vi "HandlesNullsInDB.vi"() -> ()   [LabVIEW 2019]
uses:
  <vilib>/Utility/error.llb/DialogType.ctl
  <vilib>/addons/database/Connection.llb/DB Tools Open Connec (String).vi
  <vilib>/addons/database/_DB Variant To Data/Database Variant To Data.xnode
  <vilib>/addons/database/NI_Database_API.lvlib
panel:
  out "Null Value Handled For  String":string[][](array[string])
  out "Original Data":string[][](array[string])
  out "With   Null Handled  for  Numeric":variant[][](array[variant])
  out "data":variant[][](array[variant])
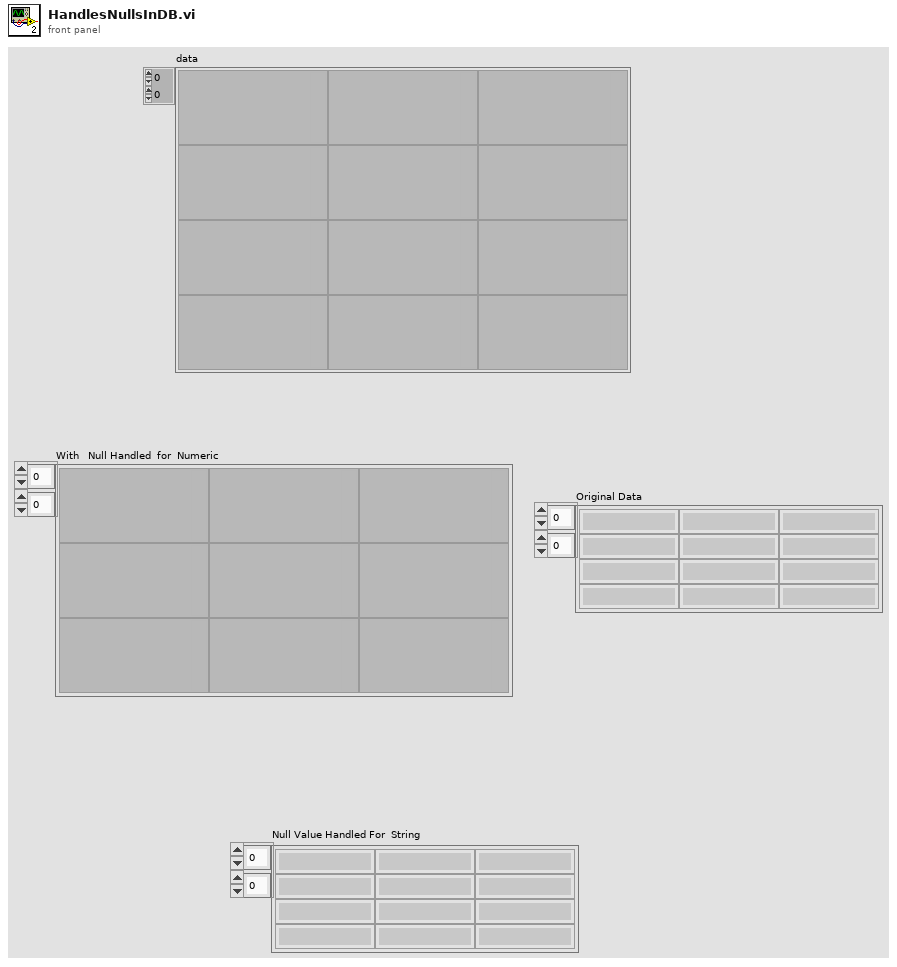
[diagram p1: front panel]
types:
  T1 = typedef "DialogType.ctl" = u16
  T2 = typedef "NI_Database_API.lvlib/Conn ObjectReference.ctl" = refnum<k1>
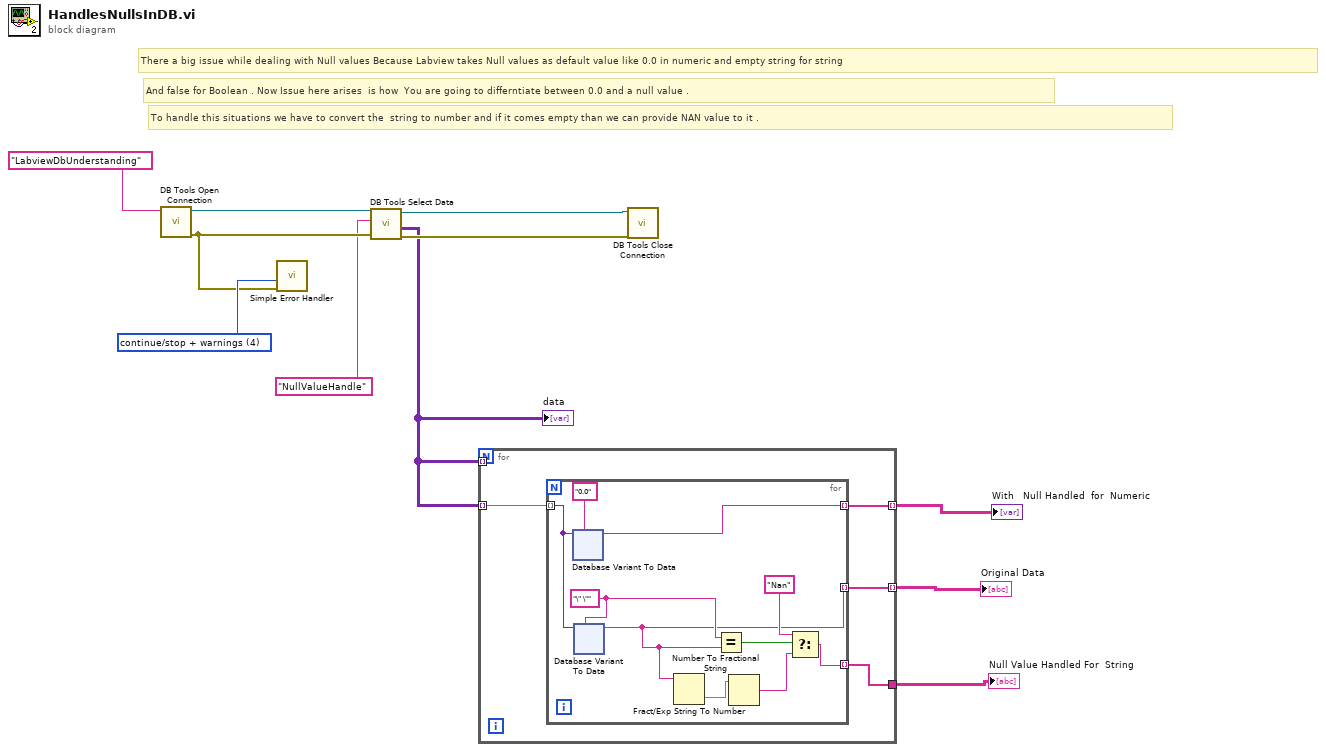
[diagram p0: block diagram]
diagram:
  w10 = T1 4 items=["no dialog", "OK message", "continue or stop message", "OK message + warnings", "continue/stop + warnings"] ("type of dialog (OK msg:1)")
  # "To handle this situations we have to convert the  string to number and if it comes empty than we can provide NAN value to it ."
  # "And false for Boolean . Now Issue here arises  is how  You are going to differntiate between 0.0 and a null value ."
  # "There a big issue while dealing with Null values Because Labview takes Null values as default value like 0.0 in numeric and empty string for string"
  n1 = call-poly <vilib>:"DB Tools Open Connection.vi"("connection information"="LabviewDbUnderstanding") -> ("error out"=w8:errorcluster, "connection reference"=w9:T2)  [unwired: 7 in]
  n2 = call <vilib>:"Simple Error Handler.vi"("type of dialog (OK msg:1)"=w10, "error in (no error)"=w8) -> ()  [unwired: 3 in, 5 out]
  n3 = call <vilib>:"DB Tools Select Data.vi"("error in (no error)"=w8, "table"="NullValueHandle", "connection reference"=w9) -> ("error out"=w5:errorcluster, "data"=w4:variant[][], "connection reference out"=w6:T2)  [unwired: 3 in]
  "data" <- w4
  n4 = for {
    tunnel: w4 -> [_] mode=indexing
    tunnel: w4 -> [w15] mode=indexing
    tunnel: [w14] -> w3 mode=indexing
    tunnel: [w13] -> w2 mode=indexing
    tunnel: [w12] -> w1 mode=indexing
    tunnel: [w12] -> _
    n5 = for {
      tunnel: w15 -> [w23] mode=indexing
      tunnel: [w25] -> w14 mode=indexing
      tunnel: [w19] -> w13 mode=indexing
      tunnel: [w16] -> w12 mode=indexing
      w22 = "\" \""
      n6 = xnode "Database Variant To Data"("database variant"=w23, "type"="0.0") -> ("data"=w25:string)  [unwired: 1 in, 1 out]
      n7 = xnode "Database Variant To Data"("database variant"=w23, "type"=w22) -> ("data"=w19:string)  [unwired: 1 in, 1 out]
      n8 = Fract/Exp String To Number(string=w19) -> (number=w17:dbl)  [unwired: 3 in, 1 out]
      n9 = Equal?(x=w22, y=w19) -> (x = y?=w20:bool)
      n10 = Number To Fractional String(number=w17) -> (F-format string=w18:string)  [unwired: 3 in]
      n11 = Select(t="Nan", s=w20, f=w18) -> (s? t:f=w16:string)
    }
  }
  "With   Null Handled  for  Numeric" <- w3
  "Original Data" <- w2
  "Null Value Handled For  String" <- w1
  n12 = call <vilib>:"DB Tools Close Connection.vi"("error in (no error)"=w5, "connection reference"=w6) -> ()  [unwired: 5 in, 1 out]
